vi "Get Data.vi"(8 "error in (no error)":errorcluster, 11 "Power Meter in":refnum<class "Power Meter.lvclass">) -> (0 "error out":errorcluster, 2 "Data Out":T1[](array[typedef]), 3 "Power Meter out":refnum<class "Power Meter.lvclass">)   [LabVIEW 2015, in "Power Meter.lvclass"]
uses:
  Power Meter.lvclass
  Power Data.ctl
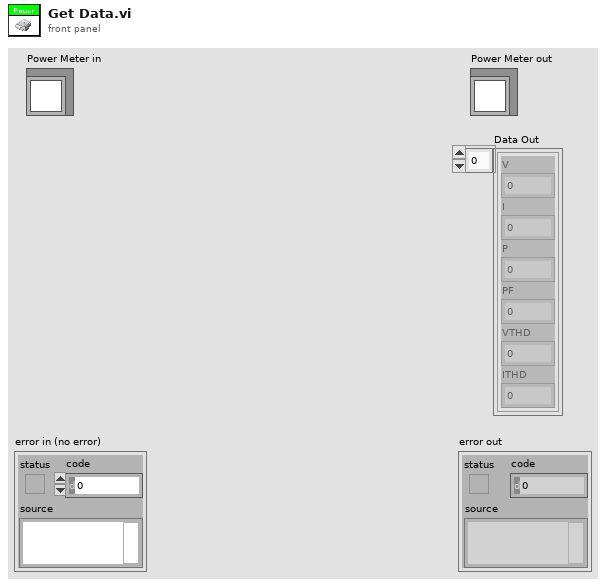
[diagram p1: front panel]
types:
  T1 = typedef "Power Meter.lvclass/Power Data.ctl" = cluster{"V":dbl, "I":dbl, "P":dbl, "PF":dbl, "VTHD":dbl, "ITHD":dbl}
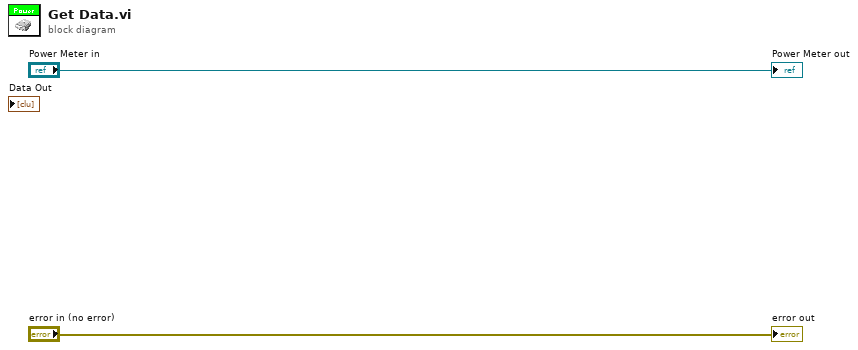
[diagram p0: block diagram]
diagram:
  "error out" <- "error in (no error)"
  "Power Meter out" <- "Power Meter in"
